vi "Framework Test.vi"() -> ()   [LabVIEW 2009]
uses:
  MyFirstTest/MyFirstTest.lvclass
  Classes/TestLoader/TestLoader.lvclass
  Classes/TextTestRunner/TextTestRunner.lvclass
panel:
  out "error out":errorcluster
  in  "verbosity (1)":u32=2
  in  "descriptions (true)":bool=TRUE
  in  "stop":bool
  out "concatenated string":string
  # "Copyright © 2007 James Kring, Inc. All rights reserved.\n\nAuthor: Jim Kring [jim.kring@jameskring.com]\n\nThis library is provided \"AS IS\" ,WITHOUT WARRANTIES OR \nCONDITIONS OF ANY KIND, either express or implied.\n\nJames Kring, Inc. -- http://www.jameskring.com"
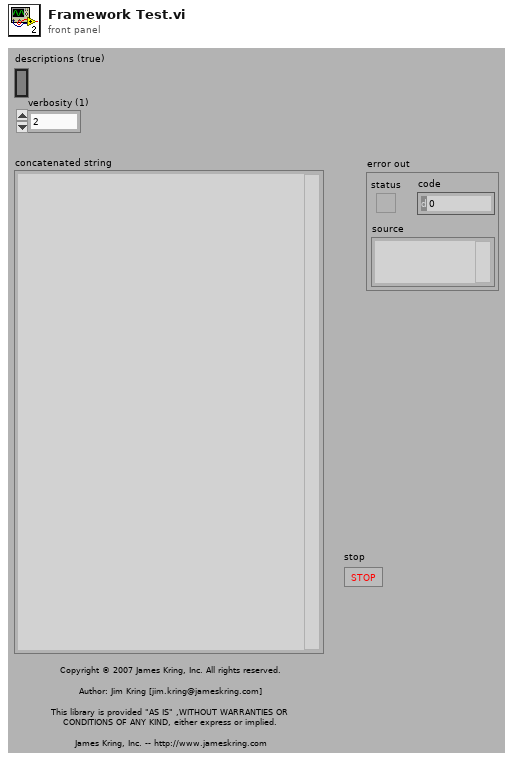
[diagram p1: front panel]
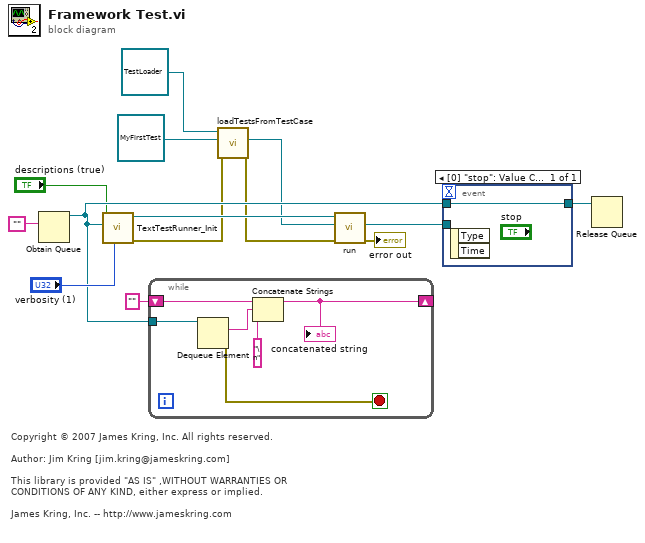
[diagram p0: block diagram]
diagram:
  # "Copyright © 2007 James Kring, Inc. All rights reserved.\n\nAuthor: Jim Kring [jim.kring@jameskring.com]\n\nThis library is provided \"AS IS\" ,WITHOUT WARRANTIES OR \nCONDITIONS OF ANY KIND, either express or implied.\n\nJames Kring, Inc. -- http://www.jameskring.com"
  n1 = Obtain Queue(element data type="") -> (queue out=w10:refnum<queue>)  [unwired: 4 in, 2 out]
  n2 = call "TextTestRunner_Init.vi"("verbosity (1)"="verbosity (1)", "descriptions (true)"="descriptions (true)", "stream"=w10) -> ("error out"=w1:errorcluster, "TextTestRunner out"=w13:refnum<class "TextTestRunner.lvclass">)  [unwired: 7 in]
  n3 = while {
    tunnel: w10 -> [w20]
    shift-right: [w17] -> _
    shift-left: "" -> [w19]
    stop <- w15 stop-if-true
    n4 = Dequeue Element(queue=w20) -> (element=w18:string, error out=w15:errorcluster)  [unwired: 2 in, 2 out]
    n5 = Concatenate Strings(w19, w18, "\n" ("string")) -> (w17:string)
    "concatenated string" <- w17
  }
  n6 = call-dynamic "loadTestsFromTestCase.vi"("error in (no error)"=w1, "TestCase"=refnum<class "MyFirstTest.lvclass"> refnum ("MyFirstTest.lvclass"), "TestLoader in"=refnum<class "TestLoader.lvclass"> refnum ("reference in")) -> ("error out"=w2:errorcluster, "TestSuite"=w3:refnum<class "TestSuite.lvclass">)  [unwired: 6 in, 1 out]
  n7 = call-dynamic "run.vi"("error in (no error)"=w2, "test"=w3, "TextTestRunner in"=w13) -> ("error out"=→"error out":errorcluster, "TextTestResults"=w6:refnum<class "_TextTestResult.lvclass">)  [unwired: 6 in, 1 out]
  n8 = event shown="[0] \"stop\": Value Change" {
    selector: _ -> [_]
    dyn-events: _ -> [_]
    timeout: _ -> [_]
    tunnel: [w21] -> w9
    tunnel: w10 -> [w21]
    tunnel: w6 -> [_]
    event [0] "stop": Value Change {
      n9 = event-data() -> ()  [unwired: 1 in, 2 out]
    }
  }
  n10 = Release Queue(queue=w9) -> ()  [unwired: 2 in, 3 out]
